vi "VI_Heat_Tape.vi"() -> ()   [LabVIEW 2019]
uses:
  <vilib>/NI/Modbus Library/API/Wrapper/Create Serial Master.vi
  <vilib>/NI/Modbus Library/API/Master/Modbus Master.lvclass
  <vilib>/NI/Modbus Library/API/Wrapper/API Main.lvlib
  <vilib>/NI/Modbus Library/Transmission Data Unit/RTU/RTU Data Unit.lvclass
panel:
  out "Value 3":sgl
  out "Value 2":sgl
  in  "Preset 2":string(combo)
  in  "Normal/Reverse Setting":string(combo)
  in  "Control Mode":string(combo)
  in  "Auto Tunning":string(combo)
  out "Connection Status":bool
  in  "?":bool
  in  "?":bool
  in  "Manual/Auto":string(combo)
  in  "Key Lock":string(combo)
  in  "Set Value":string
  in  "Preset":string(combo)
  out "Alarm Status":bool
  out "?":cluster{dbl, dbl}(graph)
  out "Heater Status":bool
  in  "Hysterisis Value":string
  out "Current Temperature Status":bool
  in  "?":bool
  out "Current Temperature (ºF)":string
  out "Heat Tape 01  Temperature (ºF)":dbl(slide) scale=65.0..85.0
  out "Value":sgl
  out "Response Message":string
  out "data string":string
  out "Query Message":string
  in  "unit ID (Defaut: 1)":u8=1
  out "Register and RAW value":u16[](array[numeric])
  in  "number of inputs (Defaut: 60)":u16
  in  "starting address (Default: 1)":u16
  in  "error check":errorcluster
  in  "Flow Control (Default: None)":u16(ring) items=["None", "XON/XOFF", "RTS/CTS", "XON/XOFF & RTS/CTS", "DTR/DSR", "XON/XOFF & DTR/DSR"]
  in  "Serial Type (Default: RTU)":enum16{"RTU", "ASCII"}(ring)
  in  "Parity (Default: None)":u16(ring)=2 items=["None", "Odd", "Even", "Mark", "Space"]
  in  "Baud Rate (Default: 115400)":u32=9600
  in  "COM Port (Default: COM7)":refnum<visa-resource-name>
  # "SpinQuest Heat Tape Temperature Monitoring System"
  # "RS-485 Connection"
  # "PXF4 Settings"
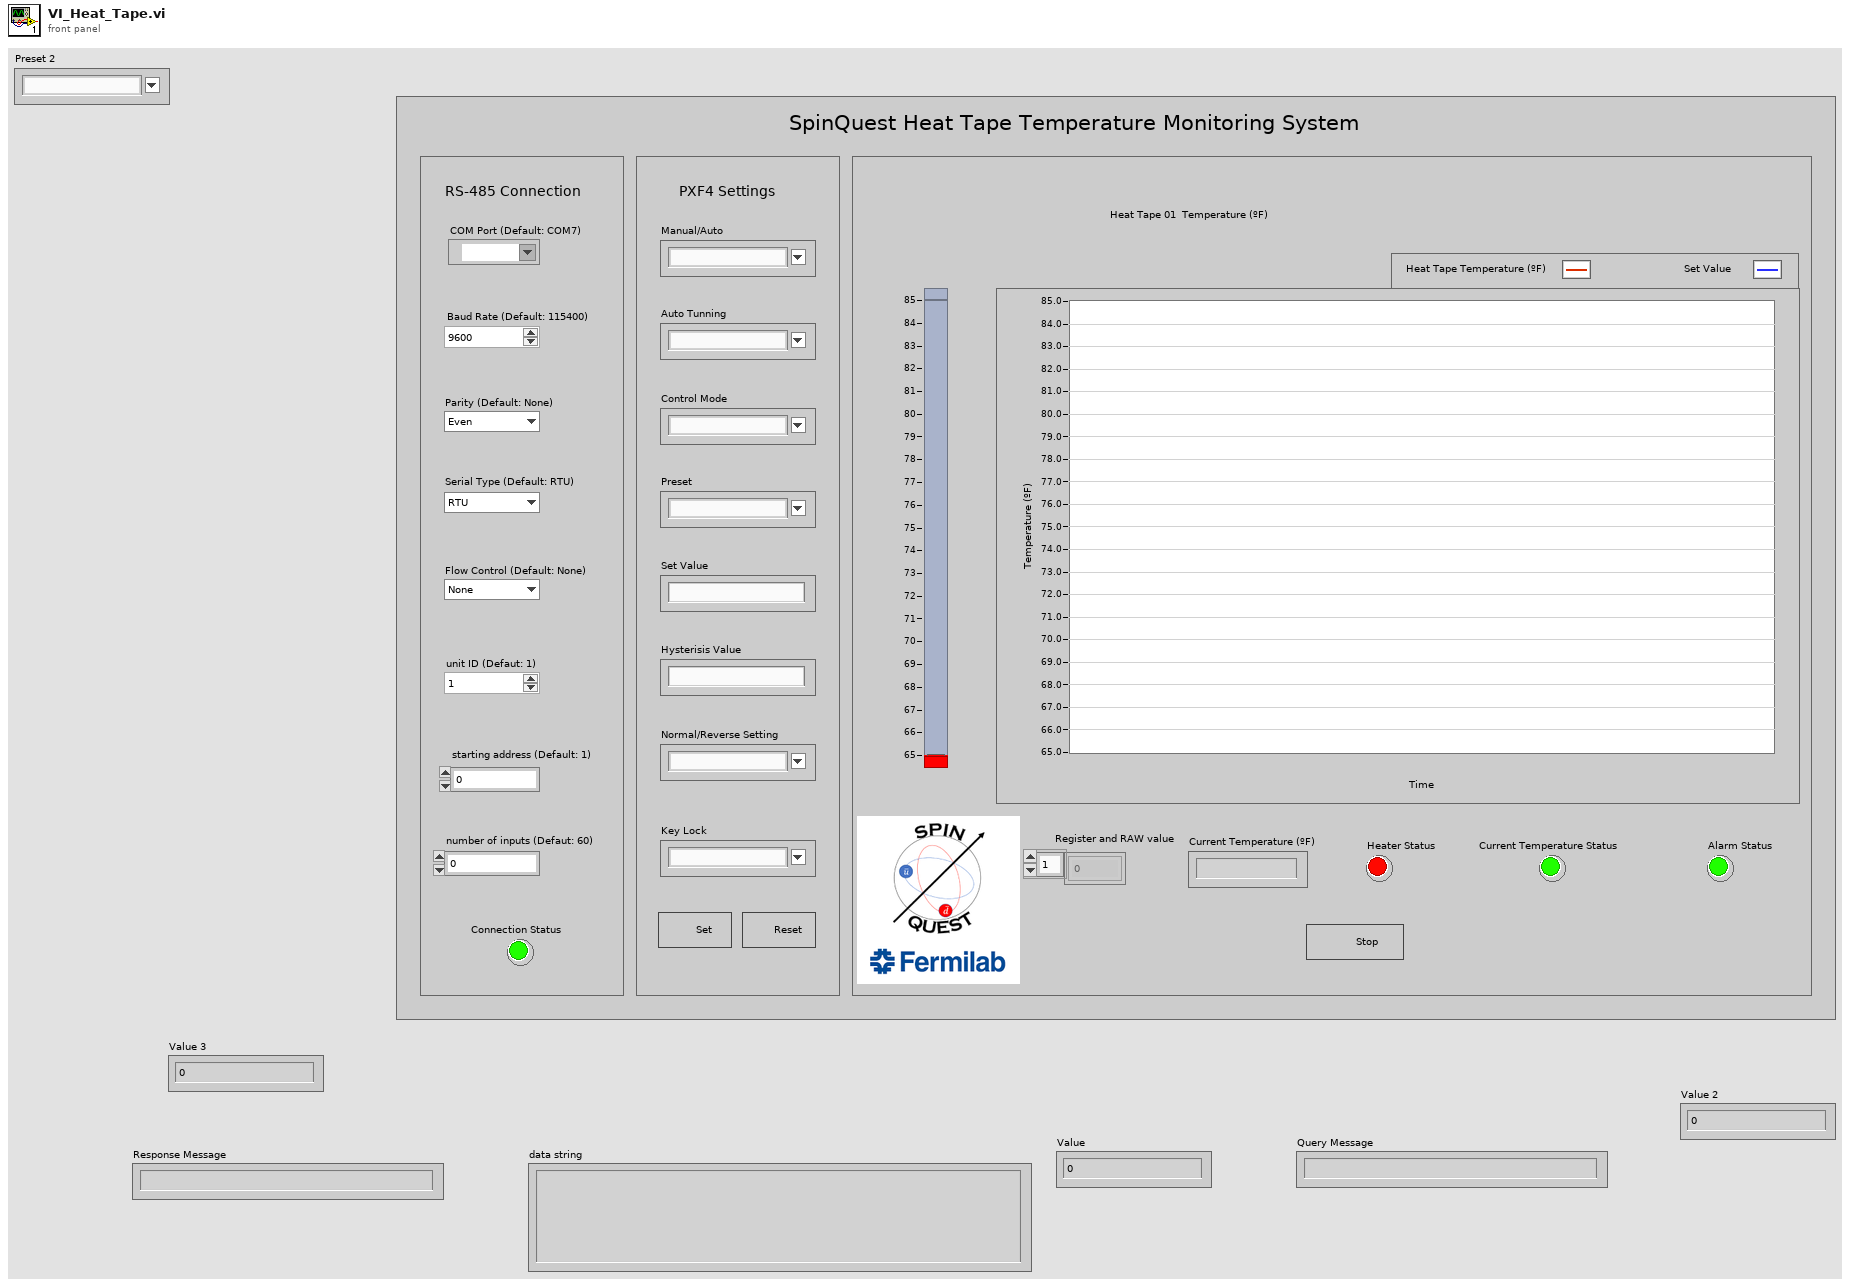
[diagram p1: front panel]
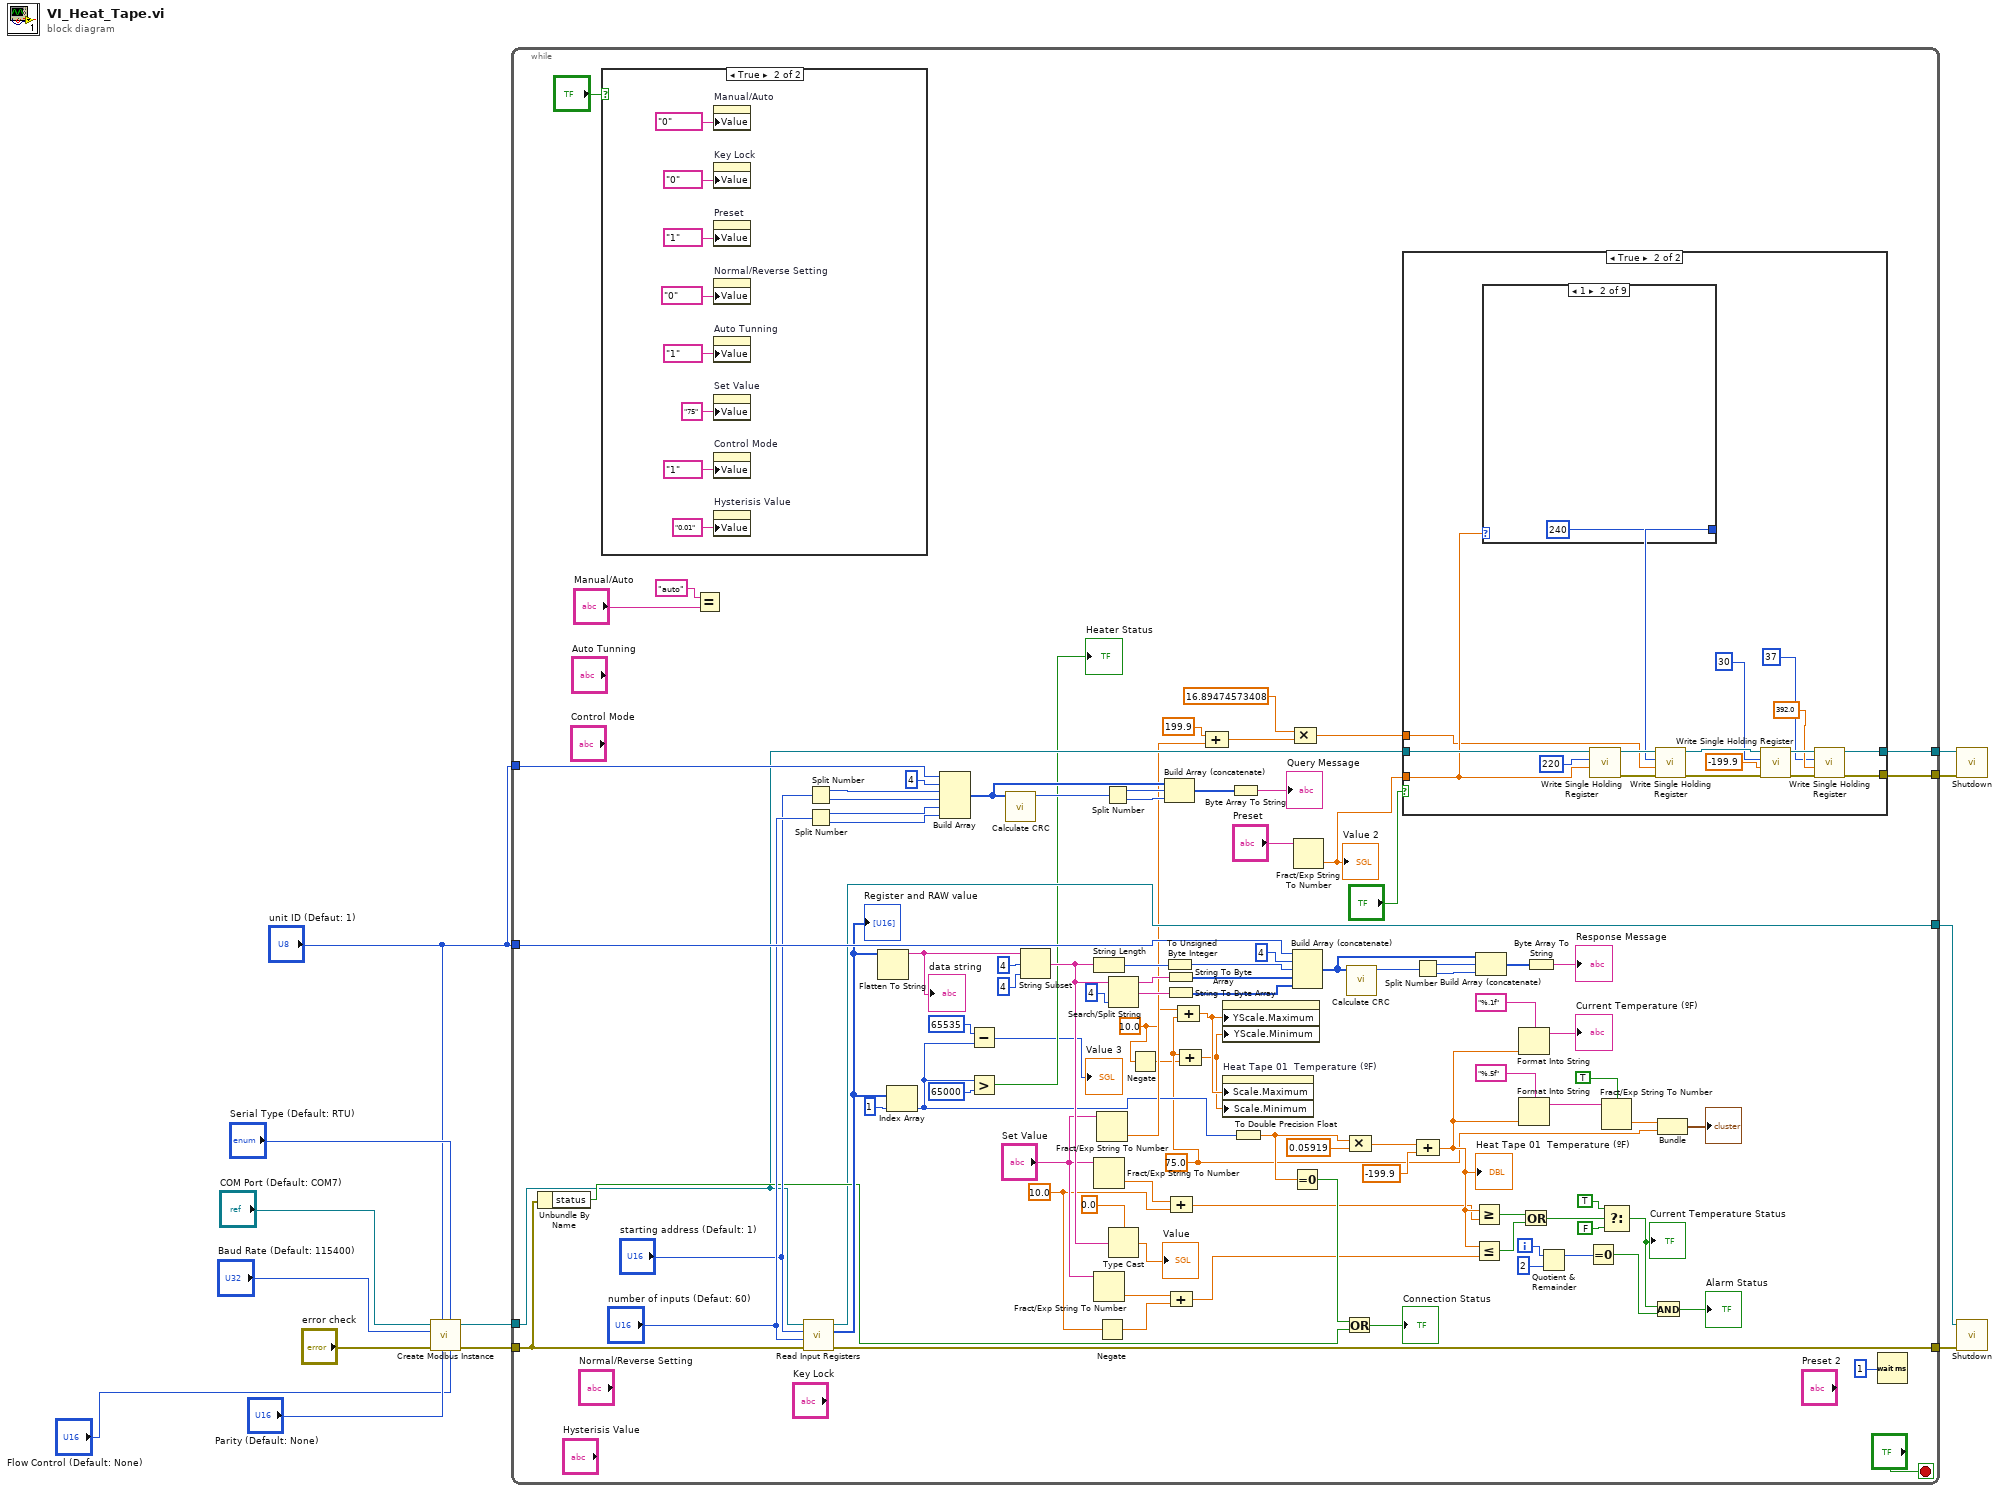
[diagram p0: block diagram]
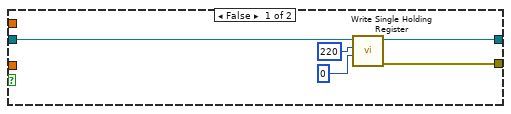
[diagram p2: hidden frame]
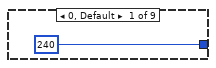
[diagram p3: hidden frame]
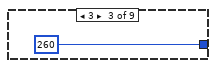
[diagram p4: hidden frame]
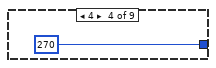
[diagram p5: hidden frame]
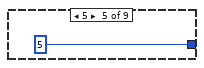
[diagram p6: hidden frame]
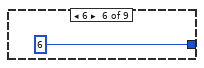
[diagram p7: hidden frame]
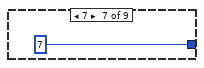
[diagram p8: hidden frame]
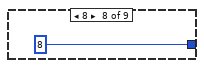
[diagram p9: hidden frame]
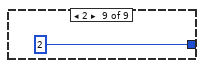
[diagram p10: hidden frame]
diagram:
  n1 = call-poly <vilib>:"Create Modbus Instance.vi"("flow control (none)"="Flow Control (Default: None)", "serial type"="Serial Type (Default: RTU)", "parity (even)"="Parity (Default: None)", "unit ID"="unit ID (Defaut: 1)", "error in"="error check", "baud rate"="Baud Rate (Default: 115400)", "VISA resource name"="COM Port (Default: COM7)") -> ("error out"=w7:errorcluster, "serial master instance"=w8:refnum<class "Modbus Master.lvclass">)  [unwired: 3 in]
  n2 = while {
    tunnel: w8 -> [w35]
    tunnel: w7 -> [w53]
    tunnel: [w54] -> w5
    tunnel: [w34] -> w3
    tunnel: "unit ID (Defaut: 1)" -> [w112]
    tunnel: "unit ID (Defaut: 1)" -> [w96]
    tunnel: [w33] -> w2
    tunnel: [w32] -> w1
    i -> [w58]
    stop <- "?" stop-if-true
    w17 = 10.0 ("value")
    w18 = 75.0 ("value")
    w38 = 10.0 ("value")
    n3 = Unbundle By Name(w53) -> ("status"=w50:bool)
    n4 = case shown="True" "?" {
      frame False {
      }
      frame True {
        n5 = property on="Manual/Auto" class="CmbBox"("Value"="0" ("Manual/Auto")) -> ()  [unwired: 2 in, 2 out]
        n6 = property on="Key Lock" class="CmbBox"("Value"="0" ("Key Lock")) -> ()  [unwired: 2 in, 2 out]
        n7 = property on="Preset" class="CmbBox"("Value"="1" ("Preset")) -> ()  [unwired: 2 in, 2 out]
        n8 = property on="Normal/Reverse Setting" class="CmbBox"("Value"="0" ("Normal/Reverse Setting")) -> ()  [unwired: 2 in, 2 out]
        n9 = property on="Auto Tunning" class="CmbBox"("Value"="1" ("Auto Tunning")) -> ()  [unwired: 2 in, 2 out]
        n10 = property on="Set Value" class="Str"("Value"="75" ("Set Value")) -> ()  [unwired: 2 in, 2 out]
        n11 = property on="Control Mode" class="CmbBox"("Value"="1" ("Control Mode")) -> ()  [unwired: 2 in, 2 out]
        n12 = property on="Hysterisis Value" class="Str"("Value"="0.01" ("Hysterisis Value")) -> ()  [unwired: 2 in, 2 out]
      }
    }
    n13 = Equal?(x="auto", y="Manual/Auto") -> ()  [unwired: 1 out]
    n14 = call-dynamic "Read Input Registers.vi"("error in"=w53, "number of inputs"="number of inputs (Defaut: 60)", "starting address"="starting address (Default: 1)", "Modbus master in"=w35) -> ("error out"=w54:errorcluster, "register values"=w75:u16[], "Modbus master out"=w34:refnum<class "Modbus Master.lvclass">)  [unwired: 5 in]
    "Register and RAW value" <- w75
    n15 = Split Number(x="starting address (Default: 1)") -> (hi(x)=w104:u8, lo(x)=w103:u8)
    n16 = Split Number(x="number of inputs (Defaut: 60)") -> (hi(x)=w102:u8, lo(x)=w101:u8)
    n17 = Flatten To String(anything=w75) -> (data string=w99:string)  [unwired: 3 in, 2 out]
    "data string" <- w99
    n18 = Index Array(array=w75, index=1) -> (element=w20:u16)
    n19 = Build Array(w112, u8 4 ("element"), w104, w103, w102, w101) -> (w110:u8[])
    n20 = Subtract(x=u16 65535 ("y"), y=w20) -> (x-y=→"Value 3":u16)
    n21 = Greater?(x=w20, y=u16 65000) -> (0:→"Heater Status":bool)
    n22 = call <vilib>:"Calculate CRC.vi"("data"=w110) -> ("CRC-16"=w109:u16)  [unwired: 10 in]
    n23 = String Subset(string=w99, offset (0)=4, length (rest)=4 ("length (rest)")) -> (substring=w83:string)
    n24 = String Length(string=w83) -> (length=w97:i32)
    n25 = Fract/Exp String To Number(string="Set Value") -> (number=w40:dbl)  [unwired: 3 in, 1 out]
    n26 = Fract/Exp String To Number(string="Set Value") -> (number=w43:dbl)  [unwired: 3 in, 1 out]
    n27 = Fract/Exp String To Number(string="Set Value") -> (number=w29:dbl)  [unwired: 3 in, 1 out]
    n28 = Negate(x=w38) -> (-x=w37:dbl)
    n29 = Split Number(x=w109) -> (hi(x)=w108:u8, lo(x)=w107:u8)
    n30 = Search/Split String(string=w83, offset (0)=4) -> (substring before match=w93:string, match + rest of string=w92:string)  [unwired: 1 in, 1 out]
    n31 = Type Cast(type=sgl 0.0, x=w83) -> (*(type *) &x=→"Value":sgl)
    n32 = Negate(x=w17) -> (-x=w16:dbl)
    n33 = Build Array (concatenate)(w110, w108, w107) -> (w106:u8[])
    n34 = To Unsigned Byte Integer(number=w97) -> (unsigned 8bit integer=w94:u8)
    n35 = String To Byte Array(string=w93) -> (unsigned byte array=w91:u8[])
    n36 = String To Byte Array(string=w92) -> (unsigned byte array=w90:u8[])
    n37 = Compound Arithmetic op=ADD(w40, w38) -> (w39:dbl)
    n38 = Compound Arithmetic op=ADD(w43, w37) -> (w42:dbl)
    n39 = Compound Arithmetic op=unknown(w17, w18) -> (w15:dbl)
    n40 = Compound Arithmetic op=unknown(w18, w16) -> (w14:dbl)
    n41 = Compound Arithmetic op=ADD(199.9 ("value"), w29) -> (w27:dbl)
    n42 = property class="WFChart (strict)"("YScale.Maximum"=w15, "YScale.Minimum"=w14) -> ()  [unwired: 2 in, 2 out]
    n43 = property on="Heat Tape 01  Temperature (ºF)" class="Slide (strict)"("Scale.Maximum"=w15, "Scale.Minimum"=w14) -> ()  [unwired: 2 in, 2 out]
    n44 = Byte Array To String(unsigned byte array=w106) -> (string=→"Query Message":string)
    n45 = To Double Precision Float(number=w20) -> (double precision float=w52:dbl)
    n46 = Build Array (concatenate)(w96, u8 4 ("element"), w94, w91, w90) -> (w84:u8[])
    n47 = Equal To 0?(x=w52) -> (x = 0?=w49:bool)
    n48 = Fract/Exp String To Number(string="Preset") -> (number=w31:dbl)  [unwired: 3 in, 1 out]
    "Value 2" <- w31
    n49 = Compound Arithmetic op=MULTIPLY(16.89474573408 ("value"), w27) -> (w25:dbl)
    n50 = Or(x=w49, y=w50) -> (x .or. y?=→"Connection Status":bool)
    n51 = call <vilib>:"Calculate CRC.vi"("data"=w84) -> ("CRC-16"=w85:u16)  [unwired: 10 in]
    n52 = Compound Arithmetic op=MULTIPLY(w52, 0.05919 ("value")) -> (w73:dbl)
    n53 = case shown="True" "?" {
      tunnel: w35 -> [w115 w134]
      tunnel: [w116 w122] -> w33
      tunnel: [w117 w121] -> w32
      tunnel: w31 -> [_ w132]
      tunnel: w25 -> [_ w129]
      frame False {
        n54 = call-dynamic "Write Single Holding Register.vi"("register to write"=u16 0, "address"=u16 220, "Modbus master in"=w115) -> ("error out"=w117:errorcluster, "Modbus master out"=w116:refnum<class "Modbus Master.lvclass">)  [unwired: 7 in]
      }
      frame True {
        n55 = case shown="1" w132 {
          tunnel: [240 240 260 270 5 6 7 8 2] -> w128
          frame 0, Default {
          }
          frame 1 {
          }
          frame 3 {
          }
          frame 4 {
          }
          frame 5 {
          }
          frame 6 {
          }
          frame 7 {
          }
          frame 8 {
          }
          frame 2 {
          }
        }
        n56 = call-dynamic "Write Single Holding Register.vi"("register to write"=w132, "address"=u16 220, "Modbus master in"=w134) -> ("error out"=w130:errorcluster, "Modbus master out"=w131:refnum<class "Modbus Master.lvclass">)  [unwired: 7 in]
        n57 = call-dynamic "Write Single Holding Register.vi"("error in"=w130, "register to write"=w129, "address"=w128, "Modbus master in"=w131) -> ("error out"=w126:errorcluster, "Modbus master out"=w127:refnum<class "Modbus Master.lvclass">)  [unwired: 6 in]
        n58 = call-dynamic "Write Single Holding Register.vi"("error in"=w126, "register to write"=-199.9 ("value"), "address"=u16 30, "Modbus master in"=w127) -> ("error out"=w124:errorcluster, "Modbus master out"=w123:refnum<class "Modbus Master.lvclass">)  [unwired: 6 in]
        n59 = call-dynamic "Write Single Holding Register.vi"("error in"=w124, "register to write"=392.0 ("value"), "address"=u16 37, "Modbus master in"=w123) -> ("error out"=w121:errorcluster, "Modbus master out"=w122:refnum<class "Modbus Master.lvclass">)  [unwired: 6 in]
      }
    }
    n60 = Split Number(x=w85) -> (hi(x)=w86:u8, lo(x)=w87:u8)
    n61 = Compound Arithmetic op=ADD(w73, -199.9 ("value")) -> (w61:dbl)
    "Heat Tape 01  Temperature (ºF)" <- w61
    n62 = Greater Or Equal?(x=w61, y=w39) -> (x >= y?=w66:bool)
    n63 = Less Or Equal?(x=w61, y=w42) -> (x <= y?=w65:bool)
    n64 = Build Array (concatenate)(w84, w86, w87) -> (w88:u8[])
    n65 = Format Into String(format string="%.1f", w61) -> (resulting string=→"Current Temperature (ºF)":string)  [unwired: 2 in, 1 out]
    n66 = Format Into String(format string="%.5f", w61) -> (resulting string=w68:string)  [unwired: 2 in, 1 out]
    n67 = Or(x=w66, y=w65) -> (x .or. y?=w64:bool)
    n68 = Byte Array To String(unsigned byte array=w88) -> (string=→"Response Message":string)
    n69 = Quotient & Remainder(x=w58, y=2) -> (x-y*floor(x/y)=w60:i32)  [unwired: 1 out]
    n70 = Equal To 0?(x=w60) -> (x = 0?=w57:bool)
    n71 = Fract/Exp String To Number(use system decimal point (T)=TRUE, string=w68) -> (number=w45:dbl)  [unwired: 2 in, 1 out]
    n72 = Select(t=TRUE, s=w64, f=FALSE) -> (s? t:f=w56:bool)
    "Current Temperature Status" <- w56
    n73 = And(x=w56, y=w57) -> (x .and. y?=→"Alarm Status":bool)
    n74 = Bundle(w45, "value"=w18) -> (→"?":cluster{dbl, "value":dbl})  [unwired: 1 in]
    n75 = Wait (ms)(milliseconds to wait=u32 1) -> ()  [unwired: 1 out]
  }
  n76 = call-dynamic "Shutdown.vi"("error in"=w1, "Modbus master in"=w2) -> ()  [unwired: 9 in, 1 out]
  n77 = call-dynamic "Shutdown.vi"("error in"=w5, "Modbus master in"=w3) -> ()  [unwired: 9 in, 1 out]
